vi "Parse OPTICAL_FLOW.vi"(11 "Data":string) -> (3 "Optical Flow Data":T1)   [LabVIEW 2014]
uses:
  Controls/MAVLink Optical Flow.ctl
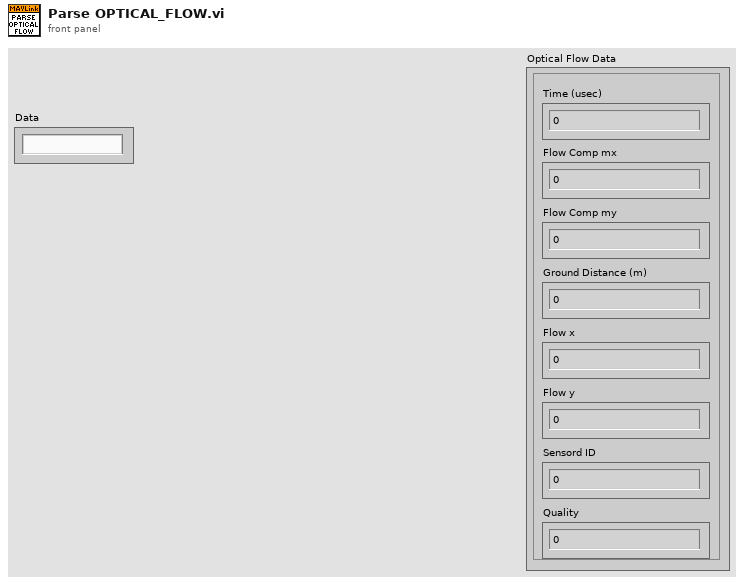
[diagram p1: front panel]
types:
  T1 = typedef "MAVLink Optical Flow.ctl" = cluster{"Time (usec)":u64, "Flow Comp mx":sgl, "Flow Comp my":sgl, "Ground Distance (m)":sgl, "Flow x":i16, "Flow y":i16, "Sensord ID":u8, "Quality":u8}
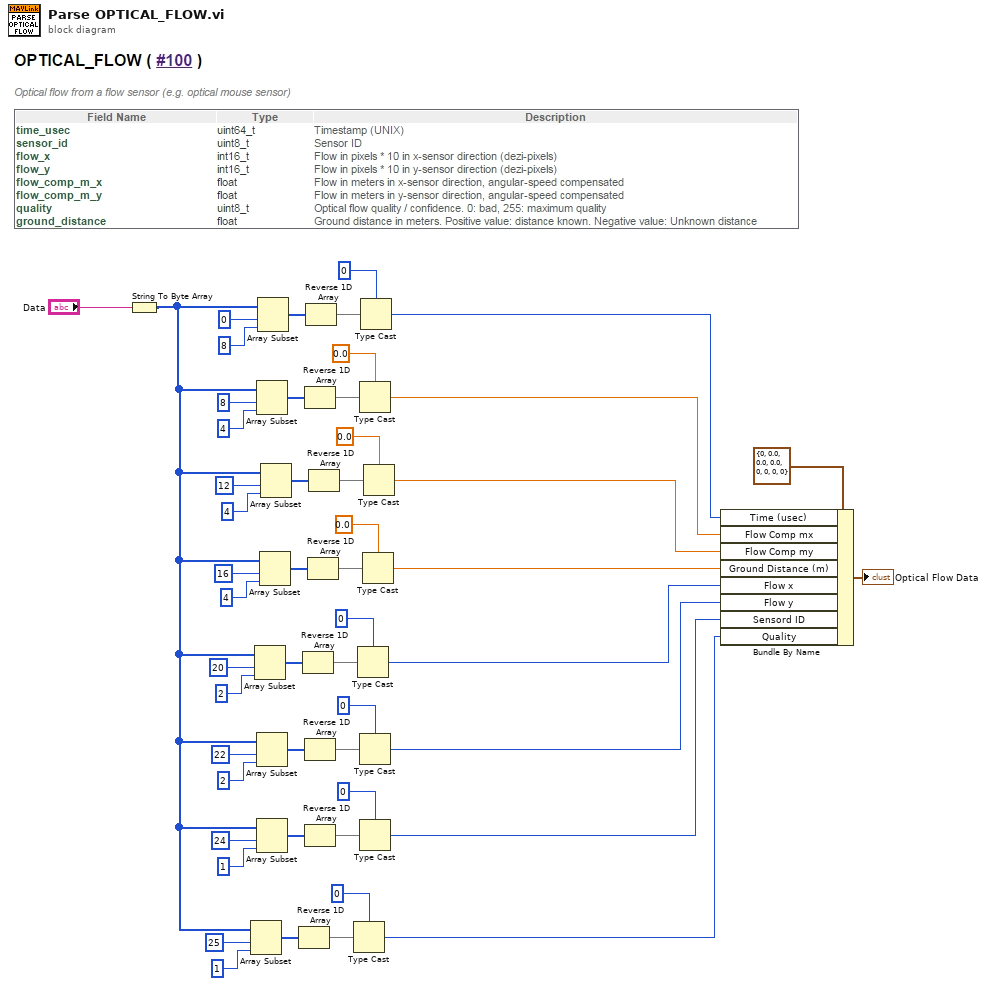
[diagram p0: block diagram]
diagram:
  n1 = String To Byte Array(string="Data") -> (unsigned byte array=w11:u8[])
  n2 = Array Subset(array=w11, index=25, length=1) -> (w13:u8[])
  n3 = Array Subset(array=w11, index=20, length=2) -> (w30:u8[])
  n4 = Array Subset(array=w11, index=8, length=4) -> (w43:u8[])
  n5 = Array Subset(array=w11, index=22, length=2) -> (w23:u8[])
  n6 = Array Subset(array=w11, index=24, length=1) -> (w20:u8[])
  n7 = Array Subset(array=w11, index=0, length=8) -> (w50:u8[])
  n8 = Array Subset(array=w11, index=16, length=4) -> (w33:u8[])
  n9 = Array Subset(array=w11, index=12, length=4) -> (w40:u8[])
  n10 = Reverse 1D Array(array=w13) -> (reversed array=w12:u8[])
  n11 = Reverse 1D Array(array=w30) -> (reversed array=w31:u8[])
  n12 = Reverse 1D Array(array=w43) -> (reversed array=w42:u8[])
  n13 = Reverse 1D Array(array=w23) -> (reversed array=w22:u8[])
  n14 = Reverse 1D Array(array=w20) -> (reversed array=w21:u8[])
  n15 = Reverse 1D Array(array=w50) -> (reversed array=w51:u8[])
  n16 = Reverse 1D Array(array=w33) -> (reversed array=w32:u8[])
  n17 = Reverse 1D Array(array=w40) -> (reversed array=w41:u8[])
  n18 = Type Cast(type=u8 0 ("single precision float"), x=w12) -> (*(type *) &x=w2:u8)
  n19 = Type Cast(type=i16 0 ("single precision float"), x=w31) -> (*(type *) &x=w5:i16)
  n20 = Type Cast(type=sgl 0.0 ("single precision float"), x=w42) -> (*(type *) &x=w8:sgl)
  n21 = Type Cast(type=i16 0 ("single precision float"), x=w22) -> (*(type *) &x=w4:i16)
  n22 = Type Cast(type=u8 0 ("single precision float"), x=w21) -> (*(type *) &x=w3:u8)
  n23 = Type Cast(type=u64 0 ("single precision float"), x=w51) -> (*(type *) &x=w9:u64)
  n24 = Type Cast(type=sgl 0.0 ("single precision float"), x=w32) -> (*(type *) &x=w6:sgl)
  n25 = Type Cast(type=sgl 0.0 ("single precision float"), x=w41) -> (*(type *) &x=w7:sgl)
  n26 = Bundle By Name(cluster=T1 {"Time (usec)"=0, "Flow Comp mx"=0.0, "Flow Comp my"=0.0, "Ground Distance (m)"=0.0, "Flow x"=0, "Flow y"=0, "Sensord ID"=0, "Quality"=0} ("Optical Flow"), "Time (usec)"=w9, "Flow Comp mx"=w8, "Flow Comp my"=w7, "Ground Distance (m)"=w6, "Flow x"=w5, "Flow y"=w4, "Sensord ID"=w3, "Quality"=w2) -> (→"Optical Flow Data":T1)
